vi "Add Time Date String + fractionsl second.vi"(9 "Prefix":string, 11 "Time in":timestamp) -> (3 "String out":string)   [LabVIEW 2012]
doc: "Adds a time-date string to incomming string"
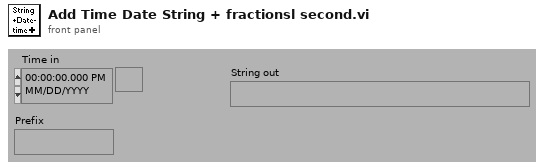
[diagram p1: front panel]
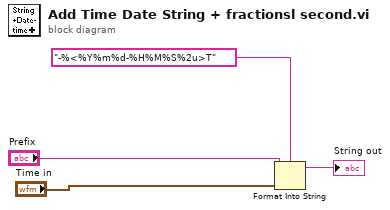
[diagram p0: block diagram]
diagram:
  n1 = Format Into String(format string="-%<%Y%m%d-%H%M%S%2u>T", initial string="Prefix", "Time in") -> (resulting string=→"String out":string)  [unwired: 1 in, 1 out]
